vi "Main Remote MSS test.vi"() -> ()   [LabVIEW 2023]
uses:
  <vilib>/ni/Actors/Network Endpoint Actors/Protocols/Network Stream Strategy/Netowrk Stream Listener/Network Stream Listener.lvclass
  MSS/Lock-In Remote Actor/Lock-In Remote Actor.lvclass
  <vilib>/ActorFramework/Actor/Actor.lvclass
panel:
  out "error out":errorcluster
  # "REMOTE"
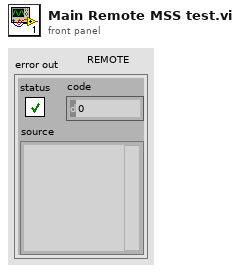
[diagram p1: front panel]
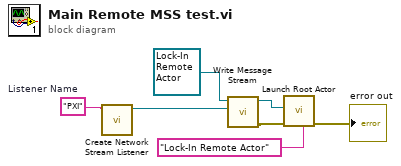
[diagram p0: block diagram]
diagram:
  w6 = "PXI"  # Listener Name
  n1 = call <vilib>:"Create Network Stream Listener.vi"("Name"=w6) -> ("Network Stream Listener"=w7:refnum<class "Network Stream Listener.lvclass">)  [unwired: 10 in]
  n2 = call "Write Message Stream.vi"("Message Stream.lvclass"=w7, "Lock-In Remote Actor in"=refnum<class "Lock-In Remote Actor.lvclass"> refnum ("Lock-In Remote Actor.lvlib:Lock-In Remote Actor.lvclass")) -> ("error out"=w5:errorcluster, "Lock-In Remote Actor out"=w2:refnum<class "Lock-In Remote Actor.lvclass">)  [unwired: 8 in]
  n3 = call <vilib>:"Launch Root Actor.vi"("Debug Alias"="Lock-In Remote Actor", "error in (no error)"=w5, "Actor"=w2) -> ("error out"=→"error out":errorcluster)  [unwired: 7 in, 1 out]
